vi "Configure.vi"(8 "error in (no error)":errorcluster caption="错误输入（无错误）", 11 "Fluke 8808A 输入":refnum<class "Fluke 8808A.lvclass">) -> (0 "error out":errorcluster caption="错误输出", 3 "Fluke 8808A 输出":refnum<class "Fluke 8808A.lvclass">)   [LabVIEW 2020, in "Fluke 8808A.lvlib" / "Fluke 8808A.lvclass"]
uses:
  Fluke 8808A.lvclass
  <instrlib>/Fluke 8808/Fluke 8808.lvlib
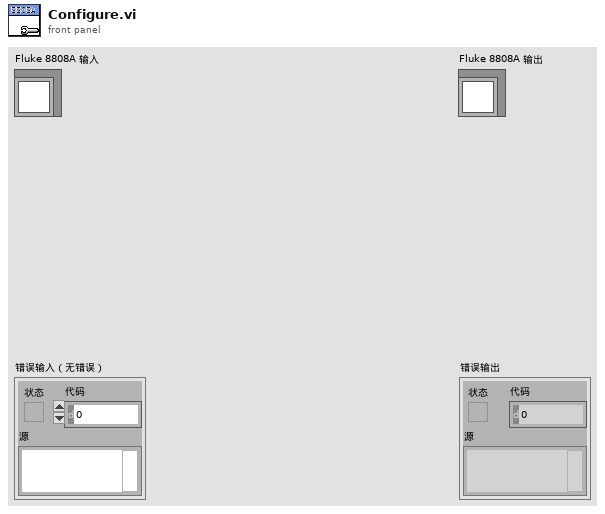
[diagram p1: front panel]
types:
  T1 = enum16{"DC Voltage", "AC Voltage", "Resistance", "DC Current", "AC Current"}
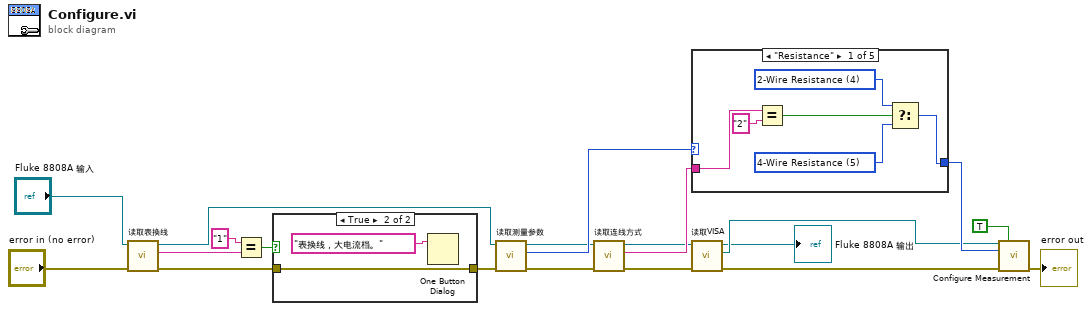
[diagram p0: block diagram]
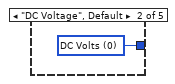
[diagram p2: hidden frame]
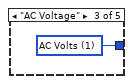
[diagram p3: hidden frame]
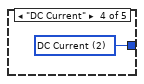
[diagram p4: hidden frame]
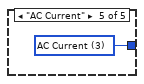
[diagram p5: hidden frame]
diagram:
  n1 = call "读取表换线.vi"("error in (no error)"="error in (no error)", "数字多用表接口输入"="Fluke 8808A 输入") -> ("error out"=w15:errorcluster, "表换线"=w13:string, "数字多用表接口输出"=w14:refnum<class "Fluke 8808A.lvclass">)  [unwired: 7 in]
  n2 = Equal?(x="1" ("y"), y=w13) -> (x = y?=w17:bool)
  n3 = case shown="True" w17 {
    tunnel: w15 -> [w21 w22]
    tunnel: [w21 w22] -> w18
    frame False {
    }
    frame True {
      n4 = One Button Dialog(message="表换线，大电流档。" ("消息")) -> ()  [unwired: 1 in, 1 out]
    }
  }
  n5 = call "读取测量参数.vi"("error in (no error)"=w18, "数字多用表接口输入"=w14) -> ("error out"=w10:errorcluster, "测量参数"=w11:T1, "数字多用表接口输出"=w9:refnum<class "Fluke 8808A.lvclass">)  [unwired: 7 in]
  n6 = call "读取连线方式.vi"("error in (no error)"=w10, "数字多用表接口输入"=w9) -> ("error out"=w7:errorcluster, "连线方式"=w8:string, "数字多用表接口输出"=w6:refnum<class "Fluke 8808A.lvclass">)  [unwired: 7 in]
  n7 = case shown="\"Resistance\"" w11 {
    tunnel: [w27 w30 w31 w32 w33] -> w12
    tunnel: w8 -> [w26 _ _ _ _]
    frame "Resistance" {
      w24 = u16 5 items=["DC Volts", "AC Volts", "DC Current", "AC Current", "2-Wire Resistance", "4-Wire Resistance", "Frequency", "AC and DC rms Current", "AC and DC rms Volts", "Continuity", "Diode"] ("Measurement Function (0: DC Volts)")
      w25 = u16 4 items=["DC Volts", "AC Volts", "DC Current", "AC Current", "2-Wire Resistance", "4-Wire Resistance", "Frequency", "AC and DC rms Current", "AC and DC rms Volts", "Continuity", "Diode"] ("Measurement Function (0: DC Volts)")
      n8 = Equal?(x=w26, y="2") -> (x = y?=w28:bool)
      n9 = Select(t=w25, s=w28, f=w24) -> (s? t:f=w27:u16)
    }
    frame "DC Voltage", Default {
      w30 = u16 0 items=["DC Volts", "AC Volts", "DC Current", "AC Current", "2-Wire Resistance", "4-Wire Resistance", "Frequency", "AC and DC rms Current", "AC and DC rms Volts", "Continuity", "Diode"] ("Measurement Function (0: DC Volts)")
    }
    frame "AC Voltage" {
      w31 = u16 1 items=["DC Volts", "AC Volts", "DC Current", "AC Current", "2-Wire Resistance", "4-Wire Resistance", "Frequency", "AC and DC rms Current", "AC and DC rms Volts", "Continuity", "Diode"] ("Measurement Function (0: DC Volts)")
    }
    frame "DC Current" {
      w32 = u16 2 items=["DC Volts", "AC Volts", "DC Current", "AC Current", "2-Wire Resistance", "4-Wire Resistance", "Frequency", "AC and DC rms Current", "AC and DC rms Volts", "Continuity", "Diode"] ("Measurement Function (0: DC Volts)")
    }
    frame "AC Current" {
      w33 = u16 3 items=["DC Volts", "AC Volts", "DC Current", "AC Current", "2-Wire Resistance", "4-Wire Resistance", "Frequency", "AC and DC rms Current", "AC and DC rms Volts", "Continuity", "Diode"] ("Measurement Function (0: DC Volts)")
    }
  }
  n10 = call "读取VISA.vi"("error in (no error)"=w7, "数字多用表接口输入"=w6) -> ("error out"=w4:errorcluster, "VISA"=w5:refnum<visa-resource-name>, "数字多用表接口输出"=→"Fluke 8808A 输出":refnum<class "Fluke 8808A.lvclass">)  [unwired: 7 in]
  n11 = call <instrlib>:"Configure Measurement.vi"("VISA resource name"=w5, "Enable Range (T: Enable)"=TRUE, "Measurement Function (0: DC Volts)"=w12, "error in (no error)"=w4) -> ("error out"=→"error out":errorcluster)  [unwired: 10 in, 1 out]
